vi "HP 33120A Function Gen - SIMPLE.vi"(8 "offset (V)":ext format="%.2f", 9 "amplitude (V)":ext=1.0 format="%.4f", 10 "frequency (Hz)":ext=1000.0 format="%.3f", 11 "Function Type":T1(ring)) -> ()   [LabVIEW 2014]
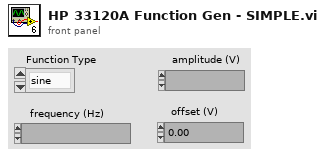
[diagram p1: front panel]
types:
  T1 = enum16{"sine", "square", "triangle", "ramp", "noise", "dc"}
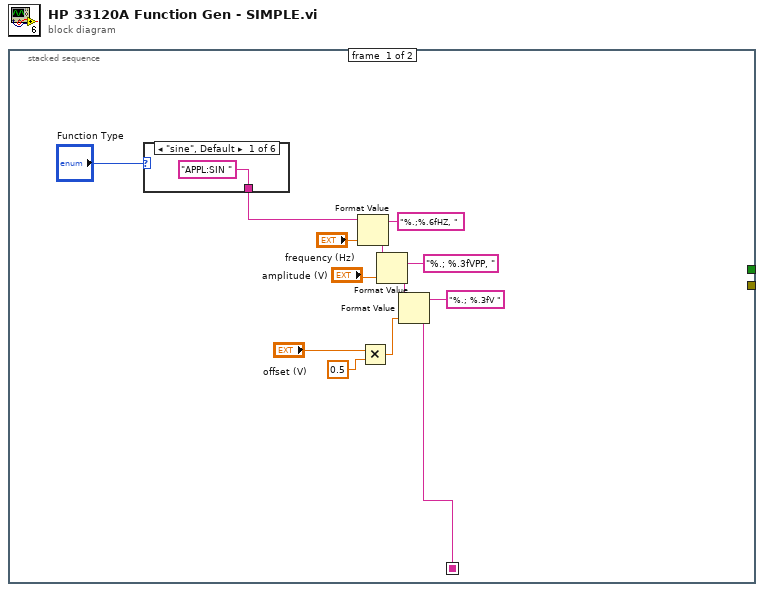
[diagram p0: block diagram]
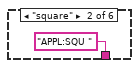
[diagram p2: hidden frame]
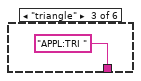
[diagram p3: hidden frame]
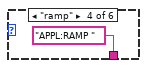
[diagram p4: hidden frame]
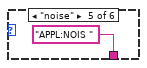
[diagram p5: hidden frame]
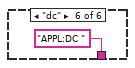
[diagram p6: hidden frame]
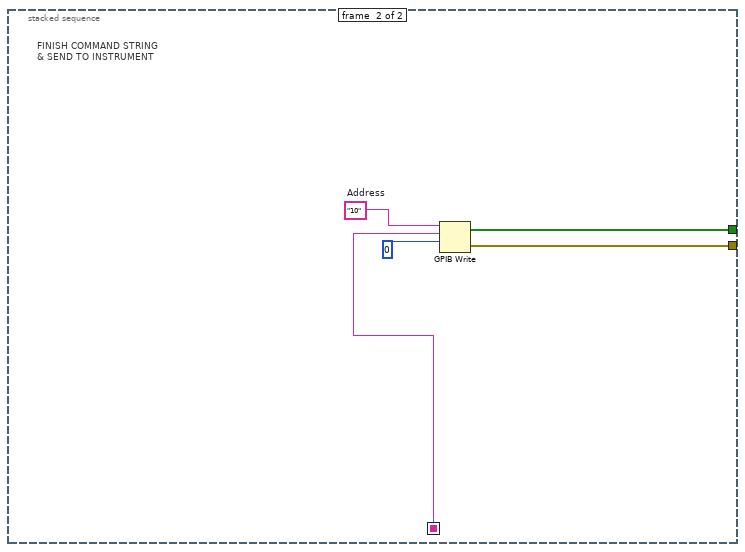
[diagram p7: hidden frame]
diagram:
  n1 = stacked-sequence {
    seq-local: [w4 _] -> [_ w20]
    tunnel: [_ w22] -> _
    tunnel: [_ w21] -> _
    frame #0 {
      n2 = case shown="\"sine\", Default" "Function Type" {
        tunnel: ["APPL:SIN " "APPL:SQU " "APPL:TRI " "APPL:RAMP " "APPL:NOIS " "APPL:DC "] -> w5
        frame "sine", Default {
        }
        frame "square" {
        }
        frame "triangle" {
        }
        frame "ramp" {
        }
        frame "noise" {
        }
        frame "dc" {
        }
      }
      n3 = Format Value(string ("")=w5, format string="%.;%.6fHZ, ", value (0)="frequency (Hz)") -> (output string=w9:string)
      n4 = Multiply(x="offset (V)", y=0.5) -> (x*y=w2:ext)
      n5 = Format Value(string ("")=w9, format string="%.; %.3fVPP, ", value (0)="amplitude (V)") -> (output string=w11:string)
      n6 = Format Value(string ("")=w11, format string="%.; %.3fV ", value (0)=w2) -> (output string=w4:string)
    }
    frame #1 {
      w23 = "10"  # Address
      # "FINISH COMMAND STRING\n& SEND TO INSTRUMENT"
      n7 = GPIB Write(0:w23, 1:w20, 2:0) -> (5:w22:bool[], 6:w21:errorcluster)  [unwired: 1 in, 1 out]
    }
  }
